vi "SFID_Send Cmd.vi"(0 "Port":refnum<visa-resource-name>, 7 "Cmd":T1="G", 11 "Error In":errorcluster) -> (4 "Port out":refnum<visa-resource-name>, 15 "Error Out":errorcluster)   [LabVIEW 2022 SP3]
uses:
  Ctls/SFID_Cmd.ctl
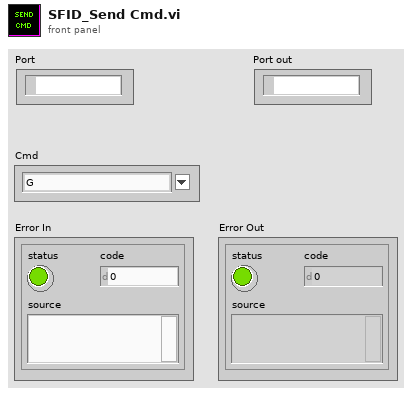
[diagram p1: front panel]
types:
  T1 = typedef "SFID_Cmd.ctl" = string
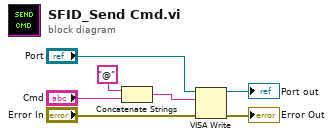
[diagram p0: block diagram]
diagram:
  n1 = Concatenate Strings("@", "Cmd") -> (w1:string)
  n2 = VISA Write(VISA resource name="Port", write buffer=w1, error in (no error)="Error In") -> (VISA resource name out=→"Port out":refnum<visa-resource-name>, error out=→"Error Out":errorcluster)  [unwired: 1 out]
